vi "CloseFile.vi"(8 "error in (no error)":errorcluster, 11 "FileHandler in":refnum<class "FileHandler.lvclass">) -> (0 "error out":errorcluster)   [LabVIEW 2021]
uses:
  Interfaces/FileHandler/FileHandler.lvclass
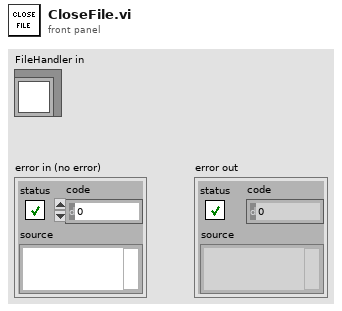
[diagram p1: front panel]
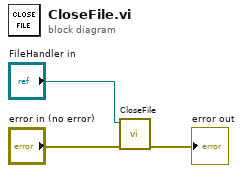
[diagram p0: block diagram]
diagram:
  n1 = call-dynamic "CloseFile.vi"("error in (no error)"="error in (no error)", "FileHandler in"="FileHandler in") -> ("error out"=→"error out":errorcluster)  [unwired: 9 in]
